vi "dvp Vi Get Timer Value.vi"(10 "pTimerValue":dbl, 11 "handle":u32) -> (2 "pTimerValue out":dbl, 3 "function return":u32(ring))   [LabVIEW 2018, in "LabViewDVPCamera.lvlib"]
doc: "LabviewDvp2Api dvpStatus dvpViGetTimerValue(dvpHandle handle, double *pTimerValue);"
uses:
  LabViewDVPCamera.lvlib
  LabViewDVPCamera/LabViewDVPCamera.dll
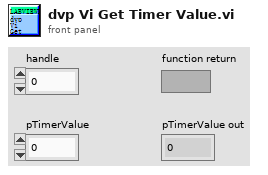
[diagram p1: front panel]
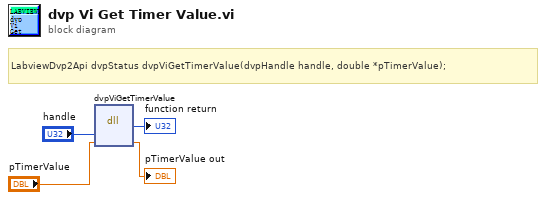
[diagram p0: block diagram]
diagram:
  # "LabviewDvp2Api dvpStatus dvpViGetTimerValue(dvpHandle handle, double *pTimerValue);"
  n1 = dll-call lib="C:/Program Files (x86)/DVP2 Labview cn 64/Sample/LabViewDVPCamera/LabViewDVPCamera.*" fn="dvpViGetTimerValue"("handle"="handle", "pTimerValue"="pTimerValue") -> (→"function return":u32, "pTimerValue"=→"pTimerValue out":dbl)  [unwired: 4 in, 2 out]
